vi "LinkSubVI.vi"(8 "error in (no error)":errorcluster, 10 "WireRef":refnum<vi>, 11 "SubVIRef In":refnum<vi>) -> (0 "error out":errorcluster, 3 "SubVIRef Out":refnum<vi>)   [LabVIEW 2011]
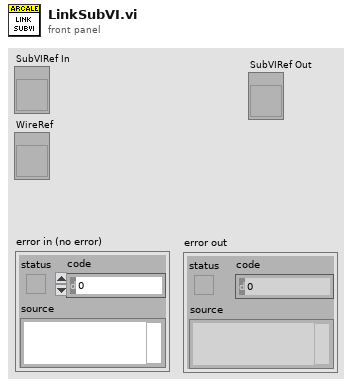
[diagram p1: front panel]
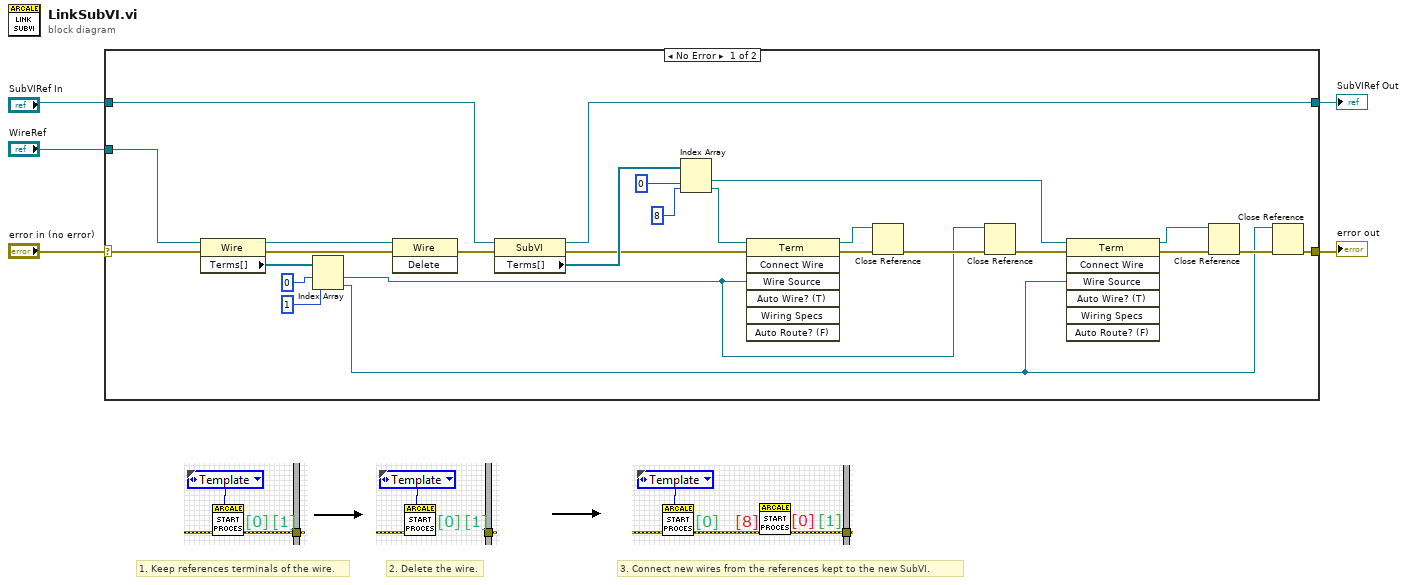
[diagram p0: block diagram]
diagram:
  # "3. Connect new wires from the references kept to the new SubVI."
  # "2. Delete the wire."
  # "1. Keep references terminals of the wire."
  n1 = case shown="No Error" "error in (no error)" {
    selector: "error in (no error)" -> [w25 w33]
    tunnel: [w12 w33] -> w4
    tunnel: "WireRef" -> [w31 _]
    tunnel: "SubVIRef In" -> [w27 w32]
    tunnel: [w16 w32] -> w1
    frame No Error {
      n2 = property class="Wire"(reference=w31, error in=w25) -> (reference out=w26:refnum<vi>, error out=w24:errorcluster, "Terms[]"=w30:refnum<vi>[])
      n3 = Index Array(array=w30, index #1=0 ("index"), index #2=1 ("index")) -> (element #1=w6:refnum<vi>, element #2=w11:refnum<vi>)
      n4 = invoke class="Wire" method="Delete"(reference=w26, error in=w24) -> (error out=w23:errorcluster)  [unwired: 1 in, 2 out]
      n5 = property class="SubVI"(reference=w27, error in=w23) -> (reference out=w16:refnum<vi>, error out=w19:errorcluster, "Terms[]"=w22:refnum<vi>[])
      n6 = Index Array(array=w22, index #1=0 ("index"), index #2=8 ("index")) -> (element #1=w17:refnum<vi>, element #2=w18:refnum<vi>)
      n7 = invoke class="Term" method="Connect Wire"(reference=w18, error in=w19, "Wire Source"=w6) -> (reference out=w7:refnum<vi>, error out=w9:errorcluster)  [unwired: 4 in, 5 out]
      n8 = Close Reference(reference=w7, error in (no error)=w9) -> (error out=w10:errorcluster)
      n9 = Close Reference(reference=w6, error in (no error)=w10) -> (error out=w8:errorcluster)
      n10 = invoke class="Term" method="Connect Wire"(reference=w17, error in=w8, "Wire Source"=w11) -> (reference out=w14:refnum<vi>, error out=w15:errorcluster)  [unwired: 4 in, 5 out]
      n11 = Close Reference(reference=w14, error in (no error)=w15) -> (error out=w13:errorcluster)
      n12 = Close Reference(reference=w11, error in (no error)=w13) -> (error out=w12:errorcluster)
    }
    frame Error {
    }
  }
  "error out" <- w4
  "SubVIRef Out" <- w1
